vi "Do.vi"(8 "error in (no error)":errorcluster, 10 "Actor in":refnum<class "Actor.lvclass">, 11 "Reply Message":refnum<class "Reply Msg.lvclass">) -> (0 "error out":errorcluster, 2 "Actor out":refnum<class "Actor.lvclass">)   [LabVIEW 2020, in "AF Specialty Messages.lvlib" / "Reply Msg.lvclass"]
uses:
  Reply Msg.lvclass
  Actor/Actor.lvclass
  Reply Msg.lvclass/Reply Msg.ctl
panel:
  in  "1122 error message":string="This actor was sent a Reply Msg. The sender set a time out duration. While this actor worked on the message, the sender timed out, resulting in this error. The Actor Framework cannot specify further what should happen; that is a policy decision that must be made by this actor. In most cases, programmers will override either this message's Do.vi or this actor's Handle Error.vi to throw away the computed result and clear this error, but some actors may do more sophisticated work (such as going ahead and sending the result to the sender in a separate asynchronous message)."
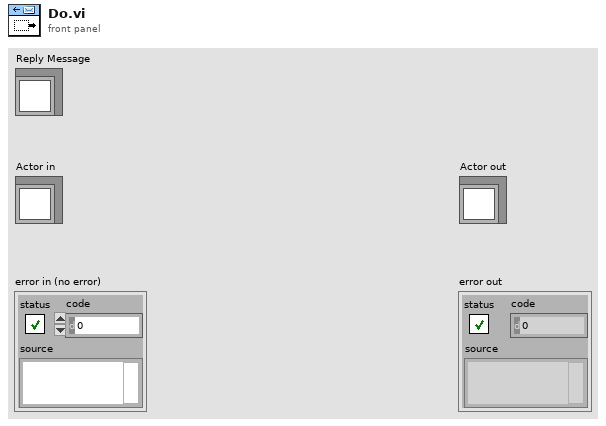
[diagram p1: front panel]
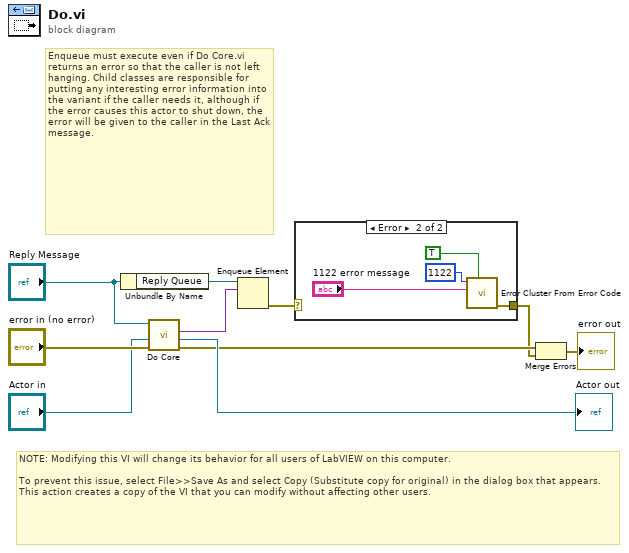
[diagram p0: block diagram]
diagram:
  # "Enqueue must execute even if Do Core.vi returns an error so that the caller is not left hanging. Child classes are responsible for putting any interesting error information into the variant if the caller needs it, although if the error causes this actor to shut down, the error will be given to the caller in the Last Ack message."
  # "NOTE: Modifying this VI will change its behavior for all users of LabVIEW on this computer.\n\nTo prevent this issue, select File>>Save As and select Copy (Substitute copy for original) in the dialog box that appears. This action creates a copy of the VI that you can modify without affecting other users."
  n1 = Unbundle By Name("Reply Message") -> ("Reply Queue"=w6:refnum<queue>)
  n2 = call-dynamic "Do Core.vi"("error in (no error)"="error in (no error)", "Actor in"="Actor in", "Reply Message"="Reply Message") -> ("error out"=w3:errorcluster, "Actor out"=→"Actor out":refnum<class "Actor.lvclass">, "Reply"=w5:variant)  [unwired: 6 in]
  n3 = Enqueue Element(queue=w6, element=w5) -> (error out=w2:errorcluster)  [unwired: 2 in, 2 out]
  n4 = case shown="Error" w2 {
    selector: w2 -> [w11 _]
    tunnel: [w11 w12] -> w1
    frame No Error {
    }
    frame Error {
      n5 = call <vilib>:"Error Cluster From Error Code.vi"("show call chain? (False)"=TRUE, "error message (\"\")"="1122 error message", "error code (0)"=1122) -> ("error out"=w12:errorcluster)  [unwired: 6 in]
    }
  }
  n6 = Merge Errors(w3, w1) -> (→"error out":errorcluster)
